vi "main.vi"() -> ()   [LabVIEW 2023] (continued)
FF\tFF\tA4\r\n      2592  1FFFFFFF   00000004    8        00\t00\tFF\tFF\tFF\tFF\tFF\tFF\r\n      2642  18F120F0   00000004    8        2B\t75\t60\tB1\tB0\t01\tFF\tFF\r\n      2641  18F11FF0   00000004    8        FF\t3F\t90\t68\t88\t1B\t10\t2C\r\n      2632  1FFFFFFF   00000004    8        00\t20\tFF\tFF\tFF\tFF\tFF\tFF\r\n      2623  0CF102A7   00000004    8        30\t75\tE0\t2E\t80\tFF\tFF\tFD\r\n      2623  0CF101A7   00000004    8        68\t00\t97\tCC\t00\t16\t39\t9D\r\n      2622  1FFFFFFF   00000004    8        00\t00\tFF\tFF\tFF\tFF\tFF\tFF\r\n      2612  1FFFFFFF   00000004    8        00\t00\tFF\tFF\tFF\tFF\tFF\tFF\r\n      2603  0CF102A7   00000004    8        30\t75\tE0\t2E\t80\tFF\tFF\tFD\r\n      2603  0CF101A7   00000004    8        68\t00\t97\tCC\t00\t16\t39\t9C\r\n      2602  1FFFFFFF   00000004    8        00\t00\tFF\tFF\tFF\tFF\tFF\tFF\r\n      2593  18F106A7   00000004    8        00\tF7\tFF\tFF\tFF\tFF\tFF\tA4\r\n      2643  0CF101A7   00000004    8        68\t00\t97\tCC\t00\t16\t39\t9E\r\n      2642  18F120F0   00000004    8        2B\t75\t60\tB1\tB0\t01\tFF\tFF\r\n      2641  18F11FF0   00000004    8        FF\t3F\t90\t68\t88\t1B\t10\t2C\r\n      2632  1FFFFFFF   00000004    8        00\t20\tFF\tFF\tFF\tFF\tFF\tFF\r\n      2623  0CF102A7   00000004    8        30\t75\tE0\t2E\t80\tFF\tFF\tFD\r\n      2623  0CF101A7   00000004    8        68\t00\t97\tCC\t00\t16\t39\t9D\r\n      2622  1FFFFFFF   00000004    8        00\t00\tFF\tFF\tFF\tFF\tFF\tFF\r\n      2612  1FFFFFFF   00000004    8        00\t00\tFF\tFF\tFF\tFF\tFF\tFF\r\n      2603  0CF102A7   00000004    8        30\t75\tE0\t2E\t80\tFF\tFF\tFD\r\n      2603  0CF101A7   00000004    8        68\t00\t97\tCC\t00\t16\t39\t9C\r\n      2602  1FFFFFFF   00000004    8        00\t00\tFF\tFF\tFF\tFF\tFF\tFF\r\n      2643  0C3C4D4A   00000004    8        BE\tFF\tFF\t7F\t18\tFF\tFF\t52\r\n      2643  0CF101A7   00000004    8        68\t00\t97\tCC\t00\t16\t39\t9E\r\n      2642  18F120F0   00000004    8        2B\t75\t60\tB1\tB0\t01\tFF\tFF\r\n      2641  18F11FF0   00000004    8        FF\t3F\t90\t68\t88\t1B\t10\t2C\r\n      2632  1FFFFFFF   00000004    8        00\t20\tFF\tFF\tFF\tFF\tFF\tFF\r\n      2623  0CF102A7   00000004    8        30\t75\tE0\t2E\t80\tFF\tFF\tFD\r\n      2623  0CF101A7   00000004    8        68\t00\t97\tCC\t00\t16\t39\t9D\r\n      2622  1FFFFFFF   00000004    8        00\t00\tFF\tFF\tFF\tFF\tFF\tFF\r\n      2612  1FFFFFFF   00000004    8        00\t00\tFF\tFF\tFF\tFF\tFF\tFF\r\n      2603  0CF102A7   00000004    8        30\t75\tE0\t2E\t80\tFF\tFF\tFD\r\n      2603  0CF101A7   00000004    8        68\t00\t97\tCC\t00\t16\t39\t9C\r\n      2644  0CF102A7   00000004    8        30\t75\tE0\t2E\t80\tFF\tFF\tFD\r\n      2643  0C3C4D4A   00000004    8        BE\tFF\tFF\t7F\t18\tFF\tFF\t52\r\n      2643  0CF101A7   00000004    8        68\t00\t97\tCC\t00\t16\t39\t9E\r\n      2642  18F120F0   00000004    8        2B\t75\t60\tB1\tB0\t01\tFF\tFF\r\n      2641  18F11FF0   00000004    8        FF\t3F\t90\t68\t88\t1B\t10\t2C\r\n      2632  1FFFFFFF   00000004    8        00\t20\tFF\tFF\tFF\tFF\tFF\tFF\r\n      2623  0CF102A7   00000004    8        30\t75\tE0\t2E\t80\tFF\tFF\tFD\r\n      2623  0CF101A7   00000004    8        68\t00\t97\tCC\t00\t16\t39\t9D\r\n      2622  1FFFFFFF   00000004    8        00\t00\tFF\tFF\tFF\tFF\tFF\tFF\r\n      2612  1FFFFFFF   00000004    8        00\t00\tFF\tFF\tFF\tFF\tFF\tFF\r\n      2603  0CF102A7   00000004    8        30\t75\tE0\t2E\t80\tFF\tFF\tFD\r\n      2644  0CF103A7   00000004    8        17\t1F\t08\t60\tB1\t1F\t08\t52\r\n      2644  0CF102A7   00000004    8        30\t75\tE0\t2E\t80\tFF\tFF\tFD\r\n      2643  0C3C4D4A   00000004    8        BE\tFF\tFF\t7F\t18\tFF\tFF\t52\r\n      2643  0CF101A7   00000004    8        68\t00\t97\tCC\t00\t16\t39\t9E\r\n      2642  18F120F0   00000004    8        2B\t75\t60\tB1\tB0\t01\tFF\tFF\r\n      2641  18F11FF0   00000004    8        FF\t3F\t90\t68\t88\t1B\t10\t2C\r\n      2632  1FFFFFFF   00000004    8        00\t20\tFF\tFF\tFF\tFF\tFF\tFF\r\n      2623  0CF102A7   00000004    8        30\t75\tE0\t2E\t80\tFF\tFF\tFD\r\n      2623  0CF101A7   00000004    8        68\t00\t97\tCC\t00\t16\t39\t9D\r\n      2622  1FFFFFFF   00000004    8        00\t00\tFF\tFF\tFF\tFF\tFF\tFF\r\n      2612  1FFFFFFF   00000004    8        00\t00\tFF\tFF\tFF\tFF\tFF\tFF\r\n      2645  0CF104A7   00000004    8        F0\t60\t22\tFC\tFF\tFF\tFF\t52\r\n      2644  0CF103A7   00000004    8        17\t1F\t08\t60\tB1\t1F\t08\t52\r\n      2644  0CF102A7   00000004    8        30\t75\tE0\t2E\t80\tFF\tFF\tFD\r\n      2643  0C3C4D4A   00000004    8        BE\tFF\tFF\t7F\t18\tFF\tFF\t52\r\n      2643  0CF101A7   00000004    8        68\t00\t97\tCC\t00\t16\t39\t9E\r\n      2642  18F120F0   00000004    8        2B\t75\t60\tB1\tB0\t01\tFF\tFF\r\n      2641  18F11FF0   00000004    8        FF\t3F\t90\t68\t88\t1B\t10\t2C\r\n      2632  1FFFFFFF   00000004    8        00\t20\tFF\tFF\tFF\tFF\tFF\tFF\r\n      2623  0CF102A7   00000004    8        30\t75\tE0\t2E\t80\tFF\tFF\tFD\r\n      2623  0CF101A7   00000004    8        68\t00\t97\tCC\t00\t16\t39\t9D\r\n      2622  1FFFFFFF   00000004    8        00\t00\tFF\tFF\tFF\tFF\tFF\tFF\r\n      2645  0CF105A7   00000004    8        94\t11\t00\t55\tFF\tFF\tFF\t21\r\n      2645  0CF104A7   00000004    8        F0\t60\t22\tFC\tFF\tFF\tFF\t52\r\n      2644  0CF103A7   00000004    8        17\t1F\t08\t60\tB1\t1F\t08\t52\r\n      2644  0CF102A7   00000004    8        30\t75\tE0\t2E\t80\tFF\tFF\tFD\r\n      2643  0C3C4D4A   00000004    8        BE\tFF\tFF\t7F\t18\tFF\tFF\t52\r\n      2643  0CF101A7   00000004    8        68\t00\t97\tCC\t00\t16\t39\t9E\r\n      2642  18F120F0   00000004    8        2B\t75\t60\tB1\tB0\t01\tFF\tFF\r\n      2641  18F11FF0   00000004    8        FF\t3F\t90\t68\t88\t1B\t10\t2C\r\n      2632  1FFFFFFF   00000004    8        00\t20\tFF\tFF\tFF\tFF\tFF\tFF\r\n      2623  0CF102A7   00000004    8        30\t75\tE0\t2E\t80\tFF\tFF\tFD\r\n      2623  0CF101A7   00000004    8        68\t00\t97\tCC\t00\t16\t39\t9D\r\n      2646  18F106A7   00000004    8        00\tF7\tFF\tFF\tFF\tFF\tFF\tA5\r\n      2645  0CF105A7   00000004    8        94\t11\t00\t55\tFF\tFF\tFF\t21\r\n      2645  0CF104A7   00000004    8        F0\t60\t22\tFC\tFF\tFF\tFF\t52\r\n      2644  0CF103A7   00000004    8        17\t1F\t08\t60\tB1\t1F\t08\t52\r\n      2644  0CF102A7   00000004    8        30\t75\tE0\t2E\t80\tFF\tFF\tFD\r\n      2643  0C3C4D4A   00000004    8        BE\tFF\tFF\t7F\t18\tFF\tFF\t52\r\n      2643  0CF101A7   00000004    8        68\t00\t97\tCC\t00\t16\t39\t9E\r\n      2642  18F120F0   00000004    8        2B\t75\t60\tB1\tB0\t01\tFF\tFF\r\n      2641  18F11FF0   00000004    8        FF\t3F\t90\t68\t88\t1B\t10\t2C\r\n      2632  1FFFFFFF   00000004    8        00\t20\tFF\tFF\tFF\tFF\tFF\tFF\r\n      2623  0CF102A7   00000004    8        30\t75\tE0\t2E\t80\tFF\tFF\tFD\r\n      2646  18F108A7   00000004    8        F0\t00\t00\tFF\tFF\tFF\tFF\t43\r\n      2646  18F106A7   00000004    8        00\tF7\tFF\tFF\tFF\tFF\tFF\tA5\r\n      2645  0CF105A7   00000004    8        94\t11\t00\t55\tFF\tFF\tFF\t21\r\n      2645  0CF104A7   00000004    8        F0\t60\t22\tFC\tFF\tFF\tFF\t52\r\n      2644  0CF103A7   00000004    8        17\t1F\t08\t60\tB1\t1F\t08\t52\r\n      2644  0CF102A7   00000004    8        30\t75\tE0\t2E\t80\tFF\tFF\tFD\r\n      2643  0C3C4D4A   00000004    8        BE\tFF\tFF\t7F\t18\tFF\tFF\t52\r\n      2643  0CF101A7   00000004    8        68\t00\t97\tCC\t00\t16\t39\t9E\r\n      2642  18F120F0   00000004    8        2B\t75\t60\tB1\tB0\t01\tFF\tFF\r\n      2641  18F11FF0   00000004    8        FF\t3F\t90\t68\t88\t1B\t10\t2C\r\n      2632  1FFFFFFF   00000004    8        00\t20\tFF\tFF\tFF\tFF\tFF\tFF\r\n      2647  18F121F0   00000004    8        09\t19\t00\t00\tFF\tFF\tB0\t01\r\n      2646  18F108A7   00000004    8        F0\t00\t00\tFF\tFF\tFF\tFF\t43\r\n      2646  18F106A7   00000004    8        00\tF7\tFF\tFF\tFF\tFF\tFF\tA5\r\n      2645  0CF105A7   00000004    8        94\t11\t00\t55\tFF\tFF\tFF\t21\r\n      2645  0CF104A7   00000004    8        F0\t60\t22\tFC\tFF\tFF\tFF\t52\r\n      2644  0CF103A7   00000004    8        17\t1F\t08\t60\tB1\t1F\t08\t52\r\n      2644  0CF102A7   00000004    8        30\t75\tE0\t2E\t80\tFF\tFF\tFD\r\n      2643  0C3C4D4A   00000004    8        BE\tFF\tFF\t7F\t18\tFF\tFF\t52\r\n      2643  0CF101A7   00000004    8        68\t00\t97\tCC\t00\t16\t39\t9E\r\n      2642  18F120F0   00000004    8        2B\t75\t60\tB1\tB0\t01\tFF\tFF\r\n      2641  18F11FF0   00000004    8        FF\t3F\t90\t68\t88\t1B\t10\t2C\r\n      2648  18FB01A7   00000004    8        FF\t1F\tFF\tFF\tFF\tFF\tFF\tFF\r\n      2647  18F121F0   00000004    8        09\t19\t00\t00\tFF\tFF\tB0\t01\r\n      2646  18F108A7   00000004    8        F0\t00\t00\tFF\tFF\tFF\tFF\t43\r\n      2646  18F106A7   00000004    8        00\tF7\tFF\tFF\tFF\tFF\tFF\tA5\r\n      2645  0CF105A7   00000004    8        94\t11\t00\t55\tFF\tFF\tFF\t21\r\n      2645  0CF104A7   00000004    8        F0\t60\t22\tFC\tFF\tFF\tFF\t52\r\n      2644  0CF103A7   00000004    8        17\t1F\t08\t60\tB1\t1F\t08\t52\r\n      2644  0CF102A7   00000004    8        30\t75\tE0\t2E\t80\tFF\tFF\tFD\r\n      2643  0C3C4D4A   00000004    8        BE\tFF\tFF\t7F\t18\tFF\tFF\t52\r\n      2643  0CF101A7   00000004    8        68\t00\t97\tCC\t00\t16\t39\t9E\r\n      2642  18F120F0   00000004    8        2B\t75\t60\tB1\tB0\t01\tFF\tFF\r\n      2648  18FEF117   00000004    8        F7\t97\tCC\tCF\tFF\tFF\tFF\tFF\r\n      2648  18FB01A7   00000004    8        FF\t1F\tFF\tFF\tFF\tFF\tFF\tFF\r\n      2647  18F121F0   00000004    8        09\t19\t00\t00\tFF\tFF\tB0\t01\r\n      2646  18F108A7   00000004    8        F0\t00\t00\tFF\tFF\tFF\tFF\t43\r\n      2646  18F106A7   00000004    8        00\tF7\tFF\tFF\tFF\tFF\tFF\tA5\r\n      2645  0CF105A7   00000004    8        94\t11\t00\t55\tFF\tFF\tFF\t21\r\n      2645  0CF104A7   00000004    8        F0\t60\t22\tFC\tFF\tFF\tFF\t52\r\n      2644  0CF103A7   00000004    8        17\t1F\t08\t60\tB1\t1F\t08\t52\r\n      2644  0CF102A7   00000004    8        30\t75\tE0\t2E\t80\tFF\tFF\tFD\r\n      2643  0C3C4D4A   00000004    8        BE\tFF\tFF\t7F\t18\tFF\tFF\t52\r\n      2643  0CF101A7   00000004    8        68\t00\t97\tCC\t00\t16\t39\t9E\r\n      2649  1FFFFFFF   00000004    8        00\t00\tFF\tFF\tFF\tFF\tFF\tFF\r\n      2648  18FEF117   00000004    8        F7\t97\tCC\tCF\tFF\tFF\tFF\tFF\r\n      2648  18FB01A7   00000004    8        FF\t1F\tFF\tFF\tFF\tFF\tFF\tFF\r\n      2647  18F121F0   00000004    8        09\t19\t00\t00\tFF\tFF\tB0\t01\r\n      2646  18F108A7   00000004    8        F0\t00\t00\tFF\tFF\tFF\tFF\t43\r\n      2646  18F106A7   00000004    8        00\tF7\tFF\tFF\tFF\tFF\tFF\tA5\r\n      2645  0CF105A7   00000004    8        94\t11\t00\t55\tFF\tFF\tFF\t21\r\n      2645  0CF104A7   00000004    8        F0\t60\t22\tFC\tFF\tFF\tFF\t52\r\n      2644  0CF103A7   00000004    8        17\t1F\t08\t60\tB1\t1F\t08\t52\r\n      2644  0CF102A7   00000004    8        30\t75\tE0\t2E\t80\tFF\tFF\tFD\r\n      2643  0C3C4D4A   00000004    8        BE\tFF\tFF\t7F\t18\tFF\tFF\t52\r\n      2652  1FFFFFFF   00000004    8        00\t00\tFF\tFF\tFF\tFF\tFF\tFF\r\n      2649  1FFFFFFF   00000004    8        00\t00\tFF\tFF\tFF\tFF\tFF\tFF\r\n      2648  18FEF117   00000004    8        F7\t97\tCC\tCF\tFF\tFF\tFF\tFF\r\n      2648  18FB01A7   00000004    8        FF\t1F\tFF\tFF\tFF\tFF\tFF\tFF\r\n      2647  18F121F0   00000004    8        09\t19\t00\t00\tFF\tFF\tB0\t01\r\n      2646  18F108A7   00000004    8        F0\t00\t00\tFF\tFF\tFF\tFF\t43\r\n      2646  18F106A7   00000004    8        00\tF7\tFF\tFF\tFF\tFF\tFF\tA5\r\n      2645  0CF105A7   00000004    8        94\t11\t00\t55\tFF\tFF\tFF\t21\r\n      2645  0CF104A7   00000004    8        F0\t60\t22\tFC\tFF\tFF\tFF\t52\r\n      2644  0CF103A7   00000004    8        17\t1F\t08\t60\tB1\t1F\t08\t52\r\n      2644  0CF102A7   00000004    8        30\t75\tE0\t2E\t80\tFF\tFF\tFD\r\n      2662  1FFFFFFF   00000004    8        00\t00\tFF\tFF\tFF\tFF\tFF\tFF\r\n      2652  1FFFFFFF   00000004    8        00\t00\tFF\tFF\tFF\tFF\tFF\tFF\r\n      2649  1FFFFFFF   00000004    8        00\t00\tFF\tFF\tFF\tFF\tFF\tFF\r\n      2648  18FEF117   00000004    8        F7\t97\tCC\tCF\tFF\tFF\tFF\tFF\r\n      2648  18FB01A7   00000004    8        FF\t1F\tFF\tFF\tFF\tFF\tFF\tFF\r\n      2647  18F121F0   00000004    8        09\t19\t00\t00\tFF\tFF\tB0\t01\r\n      2646  18F108A7   00000004    8        F0\t00\t00\tFF\tFF\tFF\tFF\t43\r\n      2646  18F106A7   00000004    8        00\tF7\tFF\tFF\tFF\tFF\tFF\tA5\r\n      2645  0CF105A7   00000004    8        94\t11\t00\t55\tFF\tFF\tFF\t21\r\n      2645  0CF104A7   00000004    8        F0\t60\t22\tFC\tFF\tFF\tFF\t52\r\n      2644  0CF103A7   00000004    8        17\t1F\t08\t60\tB1\t1F\t08\t52\r\n      2663  0CF101A7   00000004    8        68\t00\t97\tCC\t00\t16\t39\t9F\r\n      2662  1FFFFFFF   00000004    8        00\t00\tFF\tFF\tFF\tFF\tFF\tFF\r\n      2652  1FFFFFFF   00000004    8        00\t00\tFF\tFF\tFF\tFF\tFF\tFF\r\n      2649  1FFFFFFF   00000004    8        00\t00\tFF\tFF\tFF\tFF\tFF\tFF\r\n      2648  18FEF117   00000004    8        F7\t97\tCC\tCF\tFF\tFF\tFF\tFF\r\n      2648  18FB01A7   00000004    8        FF\t1F\tFF\tFF\tFF\tFF\tFF\tFF\r\n      2647  18F121F0   00000004    8        09\t19\t00\t00\tFF\tFF\tB0\t01\r\n      2646  18F108A7   00000004    8        F0\t00\t00\tFF\tFF\tFF\tFF\t43\r\n      2646  18F106A7   00000004    8        00\tF7\tFF\tFF\tFF\tFF\tFF\tA5\r\n      2645  0CF105A7   00000004    8        94\t11\t00\t55\tFF\tFF\tFF\t21\r\n      2645  0CF104A7   00000004    8        F0\t60\t22\tFC\tFF\tFF\tFF\t52\r\n      2663  0CF102A7   00000004    8        30\t75\tE0\t2E\t80\tFF\tFF\tFD\r\n      2663  0CF101A7   00000004    8        68\t00\t97\tCC\t00\t16\t39\t9F\r\n      2662  1FFFFFFF   00000004    8        00\t00\tFF\tFF\tFF\tFF\tFF\tFF\r\n      2652  1FFFFFFF   00000004    8        00\t00\tFF\tFF\tFF\tFF\tFF\tFF\r\n      2649  1FFFFFFF   00000004    8        00\t00\tFF\tFF\tFF\tFF\tFF\tFF\r\n      2648  18FEF117   00000004    8        F7\t97\tCC\tCF\tFF\tFF\tFF\tFF\r\n      2648  18FB01A7   00000004    8        FF\t1F\tFF\tFF\tFF\tFF\tFF\tFF\r\n      2647  18F121F0   00000004    8        09\t19\t00\t00\tFF\tFF\tB0\t01\r\n      2646  18F108A7   00000004    8        F0\t00\t00\tFF\tFF\tFF\tFF\t43\r\n      2646  18F106A7   00000004    8        00\tF7\tFF\tFF\tFF\tFF\tFF\tA5\r\n      2645  0CF105A7   00000004    8        94\t11\t00\t55\tFF\tFF\tFF\t21\r\n      2672  1FFFFFFF   00000004    8        00\t00\tFF\tFF\tFF\tFF\tFF\tFF\r\n      2663  0CF102A7   00000004    8        30\t75\tE0\t2E\t80\tFF\tFF\tFD\r\n      2663  0CF101A7   00000004    8        68\t00\t97\tCC\t00\t16\t39\t9F\r\n      2662  1FFFFFFF   00000004    8        00\t00\tFF\tFF\tFF\tFF\tFF\tFF\r\n      2652  1FFFFFFF   00000004    8        00\t00\tFF\tFF\tFF\tFF\tFF\tFF\r\n      2649  1FFFFFFF   00000004    8        00\t00\tFF\tFF\tFF\tFF\tFF\tFF\r\n      2648  18FEF117   00000004    8        F7\t97\tCC\tCF\tFF\tFF\tFF\tFF\r\n      2648  18FB01A7   00000004    8        FF\t1F\tFF\tFF\tFF\tFF\tFF\tFF\r\n      2647  18F121F0   00000004    8        09\t19\t00\t00\tFF\tFF\tB0\t01\r\n      2646  18F108A7   00000004    8        F0\t00\t00\tFF\tFF\tFF\tFF\t43\r\n      2646  18F106A7   00000004    8        00\tF7\tFF\tFF\tFF\tFF\tFF\tA5\r\n      2682  1FFFFFFF   00000004    8        00\t20\tFF\tFF\tFF\tFF\tFF\tFF\r\n      2672  1FFFFFFF   00000004    8        00\t00\tFF\tFF\tFF\tFF\tFF\tFF\r\n      2663  0CF102A7   00000004    8        30\t75\tE0\t2E\t80\tFF\tFF\tFD\r\n      2663  0CF101A7   00000004    8        68\t00\t97\tCC\t00\t16\t39\t9F\r\n      2662  1FFFFFFF   00000004    8        00\t00\tFF\tFF\tFF\tFF\tFF\tFF\r\n      2652  1FFFFFFF   00000004    8        00\t00\tFF\tFF\tFF\tFF\tFF\tFF\r\n      2649  1FFFFFFF   00000004    8        00\t00\tFF\tFF\tFF\tFF\tFF\tFF\r\n      2648  18FEF117   00000004    8        F7\t97\tCC\tCF\tFF\tFF\tFF\tFF\r\n      2648  18FB01A7   00000004    8        FF\t1F\tFF\tFF\tFF\tFF\tFF\tFF\r\n      2647  18F121F0   00000004    8        09\t19\t00\t00\tFF\tFF\tB0\t01\r\n      2646  18F108A7   00000004    8        F0\t00\t00\tFF\tFF\tFF\tFF\t43\r\n      2683  0CF101A7   00000004    8        68\t00\t97\tCC\t00\t16\t39\tA0\r\n      2682  1FFFFFFF   00000004    8        00\t20\tFF\tFF\tFF\tFF\tFF\tFF\r\n      2672  1FFFFFFF   00000004    8        00\t00\tFF\tFF\tFF\tFF\tFF\tFF\r\n      2663  0CF102A7   00000004    8        30\t75\tE0\t2E\t80\tFF\tFF\tFD\r\n      2663  0CF101A7   00000004    8        68\t00\t97\tCC\t00\t16\t39\t9F\r\n      2662  1FFFFFFF   00000004    8        00\t00\tFF\tFF\tFF\tFF\tFF\tFF\r\n      2652  1FFFFFFF   00000004    8        00\t00\tFF\tFF\tFF\tFF\tFF\tFF\r\n      2649  1FFFFFFF   00000004    8        00\t00\tFF\tFF\tFF\tFF\tFF\tFF\r\n      2648  18FEF117   00000004    8        F7\t97\tCC\tCF\tFF\tFF\tFF\tFF\r\n      2648  18FB01A7   00000004    8        FF\t1F\tFF\tFF\tFF\tFF\tFF\tFF\r\n      2647  18F121F0   00000004    8        09\t19\t00\t00\tFF\tFF\tB0\t01\r\n      2683  0CF102A7   00000004    8        30\t75\tE0\t2E\t80\tFF\tFF\tFD\r\n      2683  0CF101A7   00000004    8        68\t00\t97\tCC\t00\t16\t39\tA0\r\n      2682  1FFFFFFF   00000004    8        00\t20\tFF\tFF\tFF\tFF\tFF\tFF\r\n      2672  1FFFFFFF   00000004    8        00\t00\tFF\tFF\tFF\tFF\tFF\tFF\r\n      2663  0CF102A7   00000004    8        30\t75\tE0\t2E\t80\tFF\tFF\tFD\r\n      2663  0CF101A7   00000004    8        68\t00\t97\tCC\t00\t16\t39\t9F\r\n      2662  1FFFFFFF   00000004    8        00\t00\tFF\tFF\tFF\tFF\tFF\tFF\r\n      2652  1FFFFFFF   00000004    8        00\t00\tFF\tFF\tFF\tFF\tFF\tFF\r\n      2649  1FFFFFFF   00000004    8        00\t00\tFF\tFF\tFF\tFF\tFF\tFF\r\n      2648  18FEF117   00000004    8        F7\t97\tCC\tCF\tFF\tFF\tFF\tFF\r\n      2648  18FB01A7   00000004    8        FF\t1F\tFF\tFF\tFF\tFF\tFF\tFF\r\n      2692  1FFFFFFF   00000004    8        00\t00\tFF\tFF\tFF\tFF\tFF\tFF\r\n      2683  0CF102A7   00000004    8        30\t75\tE0\t2E\t80\tFF\tFF\tFD\r\n      2683  0CF101A7   00000004    8        68\t00\t97\tCC\t00\t16\t39\tA0\r\n      2682  1FFFFFFF   00000004    8        00\t20\tFF\tFF\tFF\tFF\tFF\tFF\r\n      2672  1FFFFFFF   00000004    8        00\t00\tFF\tFF\tFF\tFF\tFF\tFF\r\n      2663  0CF102A7   00000004    8        30\t75\tE0\t2E\t80\tFF\tFF\tFD\r\n      2663  0CF101A7   00000004    8        68\t00\t97\tCC\t00\t16\t39\t9F\r\n      2662  1FFFFFFF   00000004    8        00\t00\tFF\tFF\tFF\tFF\tFF\tFF\r\n      2652  1FFFFFFF   00000004    8        00\t00\tFF\tFF\tFF\tFF\tFF\tFF\r\n      2649  1FFFFFFF   00000004    8        00\t00\tFF\tFF\tFF\tFF\tFF\tFF\r\n      2648  18FEF117   00000004    8        F7\t97\tCC\tCF\tFF\tFF\tFF\tFF\r\n      2693  18F106A7   00000004    8        00\tF7\tFF\tFF\tFF\tFF\tFF\tA6\r\n      2692  1FFFFFFF   00000004    8        00\t00\tFF\tFF\tFF\tFF\tFF\tFF\r\n      2683  0CF102A7   00000004    8        30\t75\tE0\t2E\t80\tFF\tFF\tFD\r\n      2683  0CF101A7   00000004    8        68\t00\t97\tCC\t00\t16\t39\tA0\r\n      2682  1FFFFFFF   00000004    8        00\t20\tFF\tFF\tFF\tFF\tFF\tFF\r\n      2672  1FFFFFFF   00000004    8        00\t00\tFF\tFF\tFF\tFF\tFF\tFF\r\n      2663  0CF102A7   00000004    8        30\t75\tE0\t2E\t80\tFF\tFF\tFD\r\n      2663  0CF101A7   00000004    8        68\t00\t97\tCC\t00\t16\t39\t9F\r\n      2662  1FFFFFFF   00000004    8        00\t00\tFF\tFF\tFF\tFF\tFF\tFF\r\n      2652  1FFFFFFF   00000004    8        00\t00\tFF\tFF\tFF\tFF\tFF\tFF\r\n      2649  1FFFFFFF   00000004    8        00\t00\tFF\tFF\tFF\tFF\tFF\tFF\r\n      2702  1FFFFFFF   00000004    8        00\t00\tFF\tFF\tFF\tFF\tFF\tFF\r\n      2693  18F106A7   00000004    8        00\tF7\tFF\tFF\tFF\tFF\tFF\tA6\r\n      2692  1FFFFFFF   00000004    8        00\t00\tFF\tFF\tFF\tFF\tFF\tFF\r\n      2683  0CF102A7   00000004    8        30\t75\tE0\t2E\t80\tFF\tFF\tFD\r\n      2683  0CF101A7   00000004    8        68\t00\t97\tCC\t00\t16\t39\tA0\r\n      2682  1FFFFFFF   00000004    8        00\t20\tFF\tFF\tFF\tFF\tFF\tFF\r\n      2672  1FFFFFFF   00000004    8        00\t00\tFF\tFF\tFF\tFF\tFF\tFF\r\n      2663  0CF102A7   00000004    8        30\t75\tE0\t2E\t80\tFF\tFF\tFD\r\n      2663  0CF101A7   00000004    8        68\t00\t97\tCC\t00\t16\t39\t9F\r\n      2662  1FFFFFFF   00000004    8        00\t00\tFF\tFF\tFF\tFF\tFF\tFF\r\n      2652  1FFFFFFF   00000004    8        00\t00\tFF\tFF\tFF\tFF\tFF\tFF\r\n      2703  0CF101A7   00000004    8        68\t00\t97\tCC\t00\t16\t39\tA1\r\n      2702  1FFFFFFF   00000004    8        00\t00\tFF\tFF\tFF\tFF\tFF\tFF\r\n      2693  18F106A7   00000004    8        00\tF7\tFF\tFF\tFF\tFF\tFF\tA6\r\n      2692  1FFFFFFF   00000004    8        00\t00\tFF\tFF\tFF\tFF\tFF\tFF\r\n      2683  0CF102A7   00000004    8        30\t75\tE0\t2E\t80\tFF\tFF\tFD\r\n      2683  0CF101A7   00000004    8        68\t00\t97\tCC\t00\t16\t39\tA0\r\n      2682  1FFFFFFF   00000004    8        00\t20\tFF\tFF\tFF\tFF\tFF\tFF\r\n      2672  1FFFFFFF   00000004    8        00\t00\tFF\tFF\tFF\tFF\tFF\tFF\r\n      2663  0CF102A7   00000004    8        30\t75\tE0\t2E\t80\tFF\tFF\tFD\r\n      2663  0CF101A7   00000004    8        68\t00\t97\tCC\t00\t16\t39\t9F\r\n      2662  1FFFFFFF   00000004    8        00\t00\tFF\tFF\tFF\tFF\tFF\tFF\r\n      2703  0CF102A7   00000004    8        30\t75\tE0\t2E\t80\tFF\tFF\tFD\r\n      2703  0CF101A7   00000004    8        68\t00\t97\tCC\t00\t16\t39\tA1\r\n      2702  1FFFFFFF   00000004    8        00\t00\tFF\tFF\tFF\tFF\tFF\tFF\r\n      2693  18F106A7   00000004    8        00\tF7\tFF\tFF\tFF\tFF\tFF\tA6\r\n      2692  1FFFFFFF   00000004    8        00\t00\tFF\tFF\tFF\tFF\tFF\tFF\r\n      2683  0CF102A7   00000004    8        30\t75\tE0\t2E\t80\tFF\tFF\tFD\r\n      2683  0CF101A7   00000004    8        68\t00\t97\tCC\t00\t16\t39\tA0\r\n      2682  1FFFFFFF   00000004    8        00\t20\tFF\tFF\tFF\tFF\tFF\tFF\r\n      2672  1FFFFFFF   00000004    8        00\t00\tFF\tFF\tFF\tFF\tFF\tFF\r\n      2663  0CF102A7   00000004    8        30\t75\tE0\t2E\t80\tFF\tFF\tFD\r\n      2663  0CF101A7   00000004    8        68\t00\t97\tCC\t00\t16\t39\t9F\r\n      2712  1FFFFFFF   00000004    8        00\t00\tFF\tFF\tFF\tFF\tFF\tFF\r\n      2703  0CF102A7   00000004    8        30\t75\tE0\t2E\t80\tFF\tFF\tFD\r\n      2703  0CF101A7   00000004    8        68\t00\t97\tCC\t00\t16\t39\tA1\r\n      2702  1FFFFFFF   00000004    8        00\t00\tFF\tFF\tFF\tFF\tFF\tFF\r\n      2693  18F106A7   00000004    8        00\tF7\tFF\tFF\tFF\tFF\tFF\tA6\r\n      2692  1FFFFFFF   00000004    8        00\t00\tFF\tFF\tFF\tFF\tFF\tFF\r\n      2683  0CF102A7   00000004    8        30\t75\tE0\t2E\t80\tFF\tFF\tFD\r\n      2683  0CF101A7   00000004    8        68\t00\t97\tCC\t00\t16\t39\tA0\r\n      2682  1FFFFFFF   00000004    8        00\t20\tFF\tFF\tFF\tFF\tFF\tFF\r\n      2672  1FFFFFFF   00000004    8        00\t00\tFF\tFF\tFF\tFF\tFF\tFF\r\n      2663  0CF102A7   00000004    8        30\t75\tE0\t2E\t80\tFF\tFF\tFD\r\n      2722  1FFFFFFF   00000004    8        00\t00\tFF\tFF\tFF\tFF\tFF\tFF\r\n      2712  1FFFFFFF   00000004    8        00\t00\tFF\tFF\tFF\tFF\tFF\tFF\r\n      2703  0CF102A7   00000004    8        30\t75\tE0\t2E\t80\tFF\tFF\tFD\r\n      2703  0CF101A7   00000004    8        68\t00\t97\tCC\t00\t16\t39\tA1\r\n      2702  1FFFFFFF   00000004    8        00\t00\tFF\tFF\tFF\tFF\tFF\tFF\r\n      2693  18F106A7   00000004    8        00\tF7\tFF\tFF\tFF\tFF\tFF\tA6\r\n      2692  1FFFFFFF   00000004    8        00\t00\tFF\tFF\tFF\tFF\tFF\tFF\r\n      2683  0CF102A7   00000004    8        30\t75\tE0\t2E\t80\tFF\tFF\tFD\r\n      2683  0CF101A7   00000004    8        68\t00\t97\tCC\t00\t16\t39\tA0\r\n      2682  1FFFFFFF   00000004    8        00\t20\tFF\tFF\tFF\tFF\tFF\tFF\r\n      2672  1FFFFFFF   00000004    8        00\t00\tFF\tFF\tFF\tFF\tFF\tFF\r\n      2723  0CF101A7   00000004    8        68\t00\t97\tCC\t00\t16\t39\tA2\r\n      2722  1FFFFFFF   00000004    8        00\t00\tFF\tFF\tFF\tFF\tFF\tFF\r\n      2712  1FFFFFFF   00000004    8        00\t00\tFF\tFF\tFF\tFF\tFF\tFF\r\n      2703  0CF102A7   00000004    8        30\t75\tE0\t2E\t80\tFF\tFF\tFD\r\n      2703  0CF101A7   00000004    8        68\t00\t97\tCC\t00\t16\t39\tA1\r\n      2702  1FFFFFFF   00000004    8        00\t00\tFF\tFF\tFF\tFF\tFF\tFF\r\n      2693  18F106A7   00000004    8        00\tF7\tFF\tFF\tFF\tFF\tFF\tA6\r\n      2692  1FFFFFFF   00000004    8        00\t00\tFF\tFF\tFF\tFF\tFF\tFF\r\n      2683  0CF102A7   00000004    8        30\t75\tE0\t2E\t80\tFF\tFF\tFD\r\n      2683  0CF101A7   00000004    8        68\t00\t97\tCC\t00\t16\t39\tA0\r\n      2682  1FFFFFFF   00000004    8        00\t20\tFF\tFF\tFF\tFF\tFF\tFF\r\n      2723  0CF102A7   00000004    8        30\t75\tE0\t2E\t80\tFF\tFF\tFD\r\n      2723  0CF101A7   00000004    8        68\t00\t97\tCC\t00\t16\t39\tA2\r\n      2722  1FFFFFFF   00000004    8        00\t00\tFF\tFF\tFF\tFF\tFF\tFF\r\n      2712  1FFFFFFF   00000004    8        00\t00\tFF\tFF\tFF\tFF\tFF\tFF\r\n      2703  0CF102A7   00000004    8        30\t75\tE0\t2E\t80\tFF\tFF\tFD\r\n      2703  0CF101A7   00000004    8        68\t00\t97\tCC\t00\t16\t39\tA1\r\n      2702  1FFFFFFF   00000004    8        00\t00\tFF\tFF\tFF\tFF\tFF\tFF\r\n      2693  18F106A7   00000004    8        00\tF7\tFF\tFF\tFF\tFF\tFF\tA6\r\n      2692  1FFFFFFF   00000004    8        00\t00\tFF\tFF\tFF\tFF\tFF\tFF\r\n      2683  0CF102A7   00000004    8        30\t75\tE0\t2E\t80\tFF\tFF\tFD\r\n      2683  0CF101A7   00000004    8        68\t00\t97\tCC\t00\t16\t39\tA0\r\n      2732  1FFFFFFF   00000004    8        00\t00\tFF\tFF\tFF\tFF\tFF\tFF\r\n      2723  0CF102A7   00000004    8        30\t75\tE0\t2E\t80\tFF\tFF\tFD\r\n      2723  0CF101A7   00000004    8        68\t00\t97\tCC\t00\t16\t39\tA2\r\n      2722  1FFFFFFF   00000004    8        00\t00\tFF\tFF\tFF\tFF\tFF\tFF\r\n      2712  1FFFFFFF   00000004    8        00\t00\tFF\tFF\tFF\tFF\tFF\tFF\r\n      2703  0CF102A7   00000004    8        30\t75\tE0\t2E\t80\tFF\tFF\tFD\r\n      2703  0CF101A7   00000004    8        68\t00\t97\tCC\t00\t16\t39\tA1\r\n      2702  1FFFFFFF   00000004    8        00\t00\tFF\tFF\tFF\tFF\tFF\tFF\r\n      2693  18F106A7   00000004    8        00\tF7\tFF\tFF\tFF\tFF\tFF\tA6\r\n      2692  1FFFFFFF   00000004    8        00\t00\tFF\tFF\tFF\tFF\tFF\tFF\r\n      2683  0CF102A7   00000004    8        30\t75\tE0\t2E\t80\tFF\tFF\tFD\r\n      2741  18F11FF0   00000004    8        FF\t3F\t90\t68\t88\t1B\t10\t3C\r\n      2732  1FFFFFFF   00000004    8        00\t00\tFF\tFF\tFF\tFF\tFF\tFF\r\n      2723  0CF102A7   00000004    8        30\t75\tE0\t2E\t80\tFF\tFF\tFD\r\n      2723  0CF101A7   00000004    8        68\t00\t97\tCC\t00\t16\t39\tA2\r\n      2722  1FFFFFFF   00000004    8        00\t00\tFF\tFF\tFF\tFF\tFF\tFF\r\n      2712  1FFFFFFF   00000004    8        00\t00\tFF\tFF\tFF\tFF\tFF\tFF\r\n      2703  0CF102A7   00000004    8        30\t75\tE0\t2E\t80\tFF\tFF\tFD\r\n      2703  0CF101A7   00000004    8        68\t00\t97\tCC\t00\t16\t39\tA1\r\n      2702  1FFFFFFF   00000004    8        00\t00\tFF\tFF\tFF\tFF\tFF\tFF\r\n      2693  18F106A7   00000004    8        00\tF7\tFF\tFF\tFF\tFF\tFF\tA6\r\n      2692  1FFFFFFF   00000004    8        00\t00\tFF\tFF\tFF\tFF\tFF\tFF\r\n      2742  18F120F0   00000004    8        2B\t75\t60\tB1\tB0\t01\tFF\tFF\r\n      2741  18F11FF0   00000004    8        FF\t3F\t90\t68\t88\t1B\t10\t3C\r\n      2732  1FFFFFFF   00000004    8        00\t00\tFF\tFF\tFF\tFF\tFF\tFF\r\n      2723  0CF102A7   00000004    8        30\t75\tE0\t2E\t80\tFF\tFF\tFD\r\n      2723  0CF101A7   00000004    8        68\t00\t97\tCC\t00\t16\t39\tA2\r\n      2722  1FFFFFFF   00000004    8        00\t00\tFF\tFF\tFF\tFF\tFF\tFF\r\n      2712  1FFFFFFF   00000004    8        00\t00\tFF\tFF\tFF\tFF\tFF\tFF\r\n      2703  0CF102A7   00000004    8        30\t75\tE0\t2E\t80\tFF\tFF\tFD\r\n      2703  0CF101A7   00000004    8        68\t00\t97\tCC\t00\t16\t39\tA1\r\n      2702  1FFFFFFF   00000004    8        00\t00\tFF\tFF\tFF\tFF\tFF\tFF\r\n      2693  18F106A7   00000004    8        00\tF7\tFF\tFF\tFF\tFF\tFF\tA6\r\n      2743  0CF101A7   00000004    8        68\t00\t97\tCC\t00\t16\t39\tA3\r\n      2742  18F120F0   00000004    8        2B\t75\t60\tB1\tB0\t01\tFF\tFF\r\n      2741  18F11FF0   00000004    8        FF\t3F\t90\t68\t88\t1B\t10\t3C\r\n      2732  1FFFFFFF   00000004    8        00\t00\tFF\tFF\tFF\tFF\tFF\tFF\r\n      2723  0CF102A7   00000004    8        30\t75\tE0\t2E\t80\tFF\tFF\tFD\r\n      2723  0CF101A7   00000004    8        68\t00\t97\tCC\t00\t16\t39\tA2\r\n      2722  1FFFFFFF   00000004    8        00\t00\tFF\tFF\tFF\tFF\tFF\tFF\r\n      2712  1FFFFFFF   00000004    8        00\t00\tFF\tFF\tFF\tFF\tFF\tFF\r\n      2703  0CF102A7   00000004    8        30\t75\tE0\t2E\t80\tFF\tFF\tFD\r\n      2703  0CF101A7   00000004    8        68\t00\t97\tCC\t00\t16\t39\tA1\r\n      2702  1FFFFFFF   00000004    8        00\t00\tFF\tFF\tFF\tFF\tFF\tFF\r\n      2743  0C3C4D4A   00000004    8        BE\tFF\tFF\t7F\t18\tFF\tFF\t53\r\n      2743  0CF101A7   00000004    8        68\t00\t97\tCC\t00\t16\t39\tA3\r\n      2742  18F120F0   00000004    8        2B\t75\t60\tB1\tB0\t01\tFF\tFF\r\n      2741  18F11FF0   00000004    8        FF\t3F\t90\t68\t88\t1B\t10\t3C\r\n      2732  1FFFFFFF   00000004    8        00\t00\tFF\tFF\tFF\tFF\tFF\tFF\r\n      2723  0CF102A7   00000004    8        30\t75\tE0\t2E\t80\tFF\tFF\tFD\r\n      2723  0CF101A7   00000004    8        68\t00\t97\tCC\t00\t16\t39\tA2\r\n      2722  1FFFFFFF   00000004    8        00\t00\tFF\tFF\tFF\tFF\tFF\tFF\r\n      2712  1FFFFFFF   00000004    8        00\t00\tFF\tFF\tFF\tFF\tFF\tFF\r\n      2703  0CF102A7   00000004    8        30\t75\tE0\t2E\t80\tFF\tFF\tFD\r\n      2703  0CF101A7   00000004    8        68\t00\t97\tCC\t00\t16\t39\tA1\r\n      2744  0CF102A7   00000004    8        30\t75\tE0\t2E\t80\tFF\tFF\tFD\r\n      2743  0C3C4D4A   00000004    8        BE\tFF\tFF\t7F\t18\tFF\tFF\t53\r\n      2743  0CF101A7   00000004    8        68\t00\t97\tCC\t00\t16\t39\tA3\r\n      2742  18F120F0   00000004    8        2B\t75\t60\tB1\tB0\t01\tFF\tFF\r\n      2741  18F11FF0   00000004    8        FF\t3F\t90\t68\t88\t1B\t10\t3C\r\n      2732  1FFFFFFF   00000004    8        00\t00\tFF\tFF\tFF\tFF\tFF\tFF\r\n      2723  0CF102A7   00000004    8        30\t75\tE0\t2E\t80\tFF\tFF\tFD\r\n      2723  0CF101A7   00000004    8        68\t00\t97\tCC\t00\t16\t39\tA2\r\n      2722  1FFFFFFF   00000004    8        00\t00\tFF\tFF\tFF\tFF\tFF\tFF\r\n      2712  1FFFFFFF   00000004    8        00\t00\tFF\tFF\tFF\tFF\tFF\tFF\r\n      2703  0CF102A7   00000004    8        30\t75\tE0\t2E\t80\tFF\tFF\tFD\r\n      2744  0CF103A7   00000004    8        17\t1F\t08\t60\tB1\t1F\t08\t53\r\n      2744  0CF102A7   00000004    8        30\t75\tE0\t2E\t80\tFF\tFF\tFD\r\n      2743  0C3C4D4A   00000004    8        BE\tFF\tFF\t7F\t18\tFF\tFF\t53\r\n      2743  0CF101A7   00000004    8        68\t00\t97\tCC\t00\t16\t39\tA3\r\n      2742  18F120F0   00000004    8        2B\t75\t60\tB1\tB0\t01\tFF\tFF\r\n      2741  18F11FF0   00000004    8        FF\t3F\t90\t68\t88\t1B\t10\t3C\r\n      2732  1FFFFFFF   00000004    8        00\t00\tFF\tFF\tFF\tFF\tFF\tFF\r\n      2723  0CF102A7   00000004    8        30\t75\tE0\t2E\t80\tFF\tFF\tFD\r\n      2723  0CF101A7   00000004    8        68\t00\t97\tCC\t00\t16\t39\tA2\r\n      2722  1FFFFFFF   00000004    8        00\t00\tFF\tFF\tFF\tFF\tFF\tFF\r\n      2712  1FFFFFFF   00000004    8        00\t00\tFF\tFF\tFF\tFF\tFF\tFF\r\n      2745  0CF104A7   00000004    8        F0\t60\t22\tFC\tFF\tFF\tFF\t53\r\n      2744  0CF103A7   00000004    8        17\t1F\t08\t60\tB1\t1F\t08\t53\r\n      2744  0CF102A7   00000004    8        30\t75\tE0\t2E\t80\tFF\tFF\tFD\r\n      2743  0C3C4D4A   00000004    8        BE\tFF\tFF\t7F\t18\tFF\tFF\t53\r\n      2743  0CF101A7   00000004    8        68\t00\t97\tCC\t00\t16\t39\tA3\r\n      2742  18F120F0   00000004    8        2B\t75\t60\tB1\tB0\t01\tFF\tFF\r\n      2741  18F11FF0   00000004    8        FF\t3F\t90\t68\t88\t1B\t10\t3C\r\n      2732  1FFFFFFF   00000004    8        00\t00\tFF\tFF\tFF\tFF\tFF\tFF\r\n      2723  0CF102A7   00000004    8        30\t75\tE0\t2E\t80\tFF\tFF\tFD\r\n      2723  0CF101A7   00000004    8        68\t00\t97\tCC\t00\t16\t39\tA2\r\n      2722  1FFFFFFF   00000004    8        00\t00\tFF\tFF\tFF\tFF\tFF\tFF\r\n      2745  18F106A7   00000004    8        00\tF7\tFF\tFF\tFF\tFF\tFF\tA7\r\n      2745  0CF104A7   00000004    8        F0\t60\t22\tFC\tFF\tFF\tFF\t53\r\n      2744  0CF103A7   00000004    8        17\t1F\t08\t60\tB1\t1F\t08\t53\r\n      2744  0CF102A7   00000004    8        30\t75\tE0\t2E\t80\tFF\tFF\tFD\r\n      2743  0C3C4D4A   00000004    8        BE\tFF\tFF\t7F\t18\tFF\tFF\t53\r\n      2743  0CF101A7   00000004    8        68\t00\t97\tCC\t00\t16\t39\tA3\r\n      2742  18F120F0   00000004    8        2B\t75\t60\tB1\tB0\t01\tFF\tFF\r\n      2741  18F11FF0   00000004    8        FF\t3F\t90\t68\t88\t1B\t10\t3C\r\n      2732  1FFFFFFF   00000004    8        00\t00\tFF\tFF\tFF\tFF\tFF\tFF\r\n      2723  0CF102A7   00000004    8        30\t75\tE0\t2E\t80\tFF\tFF\tFD\r\n      2723  0CF101A7   00000004    8        68\t00\t97\tCC\t00\t16\t39\tA2\r\n      2746  18F121F0   00000004    8        09\t19\t00\t00\tFF\tFF\tB0\t01\r\n      2745  18F106A7   00000004    8        00\tF7\tFF\tFF\tFF\tFF\tFF\tA7\r\n      2745  0CF104A7   00000004    8        F0\t60\t22\tFC\tFF\tFF\tFF\t53\r\n      2744  0CF103A7   00000004    8        17\t1F\t08\t60\tB1\t1F\t08\t53\r\n      2744  0CF102A7   00000004    8        30\t75\tE0\t2E\t80\tFF\tFF\tFD\r\n      2743  0C3C4D4A   00000004    8        BE\tFF\tFF\t7F\t18\tFF\tFF\t53\r\n      2743  0CF101A7   00000004    8        68\t00\t97\tCC\t00\t16\t39\tA3\r\n      2742  18F120F0   00000004    8        2B\t75\t60\tB1\tB0\t01\tFF\tFF\r\n      2741  18F11FF0   00000004    8        FF\t3F\t90\t68\t88\t1B\t10\t3C\r\n      2732  1FFFFFFF   00000004    8        00\t00\tFF\tFF\tFF\tFF\tFF\tFF\r\n      2723  0CF102A7   00000004    8        30\t75\tE0\t2E\t80\tFF\tFF\tFD\r\n      2747  1FFFFFFF   00000004    8        00\t00\tFF\tFF\tFF\tFF\tFF\tFF\r\n      2746  18F121F0   00000004    8        09\t19\t00\t00\tFF\tFF\tB0\t01\r\n      2745  18F106A7   00000004    8        00\tF7\tFF\tFF\tFF\tFF\tFF\tA7\r\n      2745  0CF104A7   00000004    8        F0\t60\t22\tFC\tFF\tFF\tFF\t53\r\n      2744  0CF103A7   00000004    8        17\t1F\t08\t60\tB1\t1F\t08\t53\r\n      2744  0CF102A7   00000004    8        30\t75\tE0\t2E\t80\tFF\tFF\tFD\r\n      2743  0C3C4D4A   00000004    8        BE\tFF\tFF\t7F\t18\tFF\tFF\t53\r\n      2743  0CF101A7   00000004    8        68\t00\t97\tCC\t00\t16\t39\tA3\r\n      2742  18F120F0   00000004    8        2B\t75\t60\tB1\tB0\t01\tFF\tFF\r\n      2741  18F11FF0   00000004    8        FF\t3F\t90\t68\t88\t1B\t10\t3C\r\n      2732  1FFFFFFF   00000004    8        00\t00\tFF\tFF\tFF\tFF\tFF\tFF\r\n      2752  1FFFFFFF   00000004    8        00\t00\tFF\tFF\tFF\tFF\tFF\tFF\r\n      2747  1FFFFFFF   00000004    8        00\t00\tFF\tFF\tFF\tFF\tFF\tFF\r\n      2746  18F121F0   00000004    8        09\t19\t00\t00\tFF\tFF\tB0\t01\r\n      2745  18F106A7   00000004    8        00\tF7\tFF\tFF\tFF\tFF\tFF\tA7\r\n      2745  0CF104A7   00000004    8        F0\t60\t22\tFC\tFF\tFF\tFF\t53\r\n      2744  0CF103A7   00000004    8        17\t1F\t08\t60\tB1\t1F\t08\t53\r\n      2744  0CF102A7   00000004    8        30\t75\tE0\t2E\t80\tFF\tFF\tFD\r\n      2743  0C3C4D4A   00000004    8        BE\tFF\tFF\t7F\t18\tFF\tFF\t53\r\n      2743  0CF101A7   00000004    8        68\t00\t97\tCC\t00\t16\t39\tA3\r\n      2742  18F120F0   00000004    8        2B\t75\t60\tB1\tB0\t01\tFF\tFF\r\n      2741  18F11FF0   00000004    8        FF\t3F\t90\t68\t88\t1B\t10\t3C\r\n      2762  1FFFFFFF   00000004    8        00\t00\tFF\tFF\tFF\tFF\tFF\tFF\r\n      2752  1FFFFFFF   00000004    8        00\t00\tFF\tFF\tFF\tFF\tFF\tFF\r\n      2747  1FFFFFFF   00000004    8        00\t00\tFF\tFF\tFF\tFF\tFF\tFF\r\n      2746  18F121F0   00000004    8        09\t19\t00\t00\tFF\tFF\tB0\t01\r\n      2745  18F106A7   00000004    8        00\tF7\tFF\tFF\tFF\tFF\tFF\tA7\r\n      2745  0CF104A7   00000004    8        F0\t60\t22\tFC\tFF\tFF\tFF\t53\r\n      2744  0CF103A7   00000004    8        17\t1F\t08\t60\tB1\t1F\t08\t53\r\n      2744  0CF102A7   00000004    8        30\t75\tE0\t2E\t80\tFF\tFF\tFD\r\n      2743  0C3C4D4A   00000004    8        BE\tFF\tFF\t7F\t18\tFF\tFF\t53\r\n      2743  0CF101A7   00000004    8        68\t00\t97\tCC\t00\t16\t39\tA3\r\n      2742  18F120F0   00000004    8        2B\t75\t60\tB1\tB0\t01\tFF\tFF\r\n      2763  0CF101A7   00000004    8        68\t00\t97\tCC\t00\t16\t39\tA4\r\n      2762  1FFFFFFF   00000004    8        00\t00\tFF\tFF\tFF\tFF\tFF\tFF\r\n      2752  1FFFFFFF   00000004    8        00\t00\tFF\tFF\tFF\tFF\tFF\tFF\r\n      2747  1FFFFFFF   00000004    8        00\t00\tFF\tFF\tFF\tFF\tFF\tFF\r\n      2746  18F121F0   00000004    8        09\t19\t00\t00\tFF\tFF\tB0\t01\r\n      2745  18F106A7   00000004    8        00\tF7\tFF\tFF\tFF\tFF\tFF\tA7\r\n      2745  0CF104A7   00000004    8        F0\t60\t22\tFC\tFF\tFF\tFF\t53\r\n      2744  0CF103A7   00000004    8        17\t1F\t08\t60\tB1\t1F\t08\t53\r\n      2744  0CF102A7   00000004    8        30\t75\tE0\t2E\t80\tFF\tFF\tFD\r\n      2743  0C3C4D4A   00000004    8        BE\tFF\tFF\t7F\t18\tFF\tFF\t53\r\n      2743  0CF101A7   00000004    8        68\t00\t97\tCC\t00\t16\t39\tA3\r\n      2763  0CF102A7   00000004    8        30\t75\tE0\t2E\t80\tFF\tFF\tFD\r\n      2763  0CF101A7   00000004    8        68\t00\t97\tCC\t00\t16\t39\tA4\r\n      2762  1FFFFFFF   00000004    8        00\t00\tFF\tFF\tFF\tFF\tFF\tFF\r\n      2752  1FFFFFFF   00000004    8        00\t00\tFF\tFF\tFF\tFF\tFF\tFF\r\n      2747  1FFFFFFF   00000004    8        00\t00\tFF\tFF\tFF\tFF\tFF\tFF\r\n      2746  18F121F0   00000004    8        09\t19\t00\t00\tFF\tFF\tB0\t01\r\n      2745  18F106A7   00000004    8        00\tF7\tFF\tFF\tFF\tFF\tFF\tA7\r\n      2745  0CF104A7   00000004    8        F0\t60\t22\tFC\tFF\tFF\tFF\t53\r\n      2744  0CF103A7   00000004    8        17\t1F\t08\t60\tB1\t1F\t08\t53\r\n      2744  0CF102A7   00000004    8        30\t75\tE0\t2E\t80\tFF\tFF\tFD\r\n      2743  0C3C4D4A   00000004    8        BE\tFF\tFF\t7F\t18\tFF\tFF\t53\r\n      2772  1FFFFFFF   00000004    8        00\t00\tFF\tFF\tFF\tFF\tFF\tFF\r\n      2763  0CF102A7   00000004    8        30\t75\tE0\t2E\t80\tFF\tFF\tFD\r\n      2763  0CF101A7   00000004    8        68\t00\t97\tCC\t00\t16\t39\tA4\r\n      2762  1FFFFFFF   00000004    8        00\t00\tFF\tFF\tFF\tFF\tFF\tFF\r\n      2752  1FFFFFFF   00000004    8        00\t00\tFF\tFF\tFF\tFF\tFF\tFF\r\n      2747  1FFFFFFF   00000004    8        00\t00\tFF\tFF\tFF\tFF\tFF\tFF\r\n      2746  18F121F0   00000004    8        09\t19\t00\t00\tFF\tFF\tB0\t01\r\n      2745  18F106A7   00000004    8        00\tF7\tFF\tFF\tFF\tFF\tFF\tA7\r\n      2745  0CF104A7   00000004    8        F0\t60\t22\tFC\tFF\tFF\tFF\t53\r\n      2744  0CF103A7   00000004    8        17\t1F\t08\t60\tB1\t1F\t08\t53\r\n      2744  0CF102A7   00000004    8        30\t75\tE0\t2E\t80\tFF\tFF\tFD\r\n      2782  1FFFFFFF   00000004    8        00\t00\tFF\tFF\tFF\tFF\tFF\tFF\r\n      2772  1FFFFFFF   00000004    8        00\t00\tFF\tFF\tFF\tFF\tFF\tFF\r\n      2763  0CF102A7   00000004    8        30\t75\tE0\t2E\t80\tFF\tFF\tFD\r\n      2763  0CF101A7   00000004    8        68\t00\t97\tCC\t00\t16\t39\tA4\r\n      2762  1FFFFFFF   00000004    8        00\t00\tFF\tFF\tFF\tFF\tFF\tFF\r\n      2752  1FFFFFFF   00000004    8        00\t00\t
